vi "log.vi"(9 "响应":string, 11 "发送":string) -> ()   [LabVIEW 2015]
panel:
  in  "应用程序输入":refnum<vi>
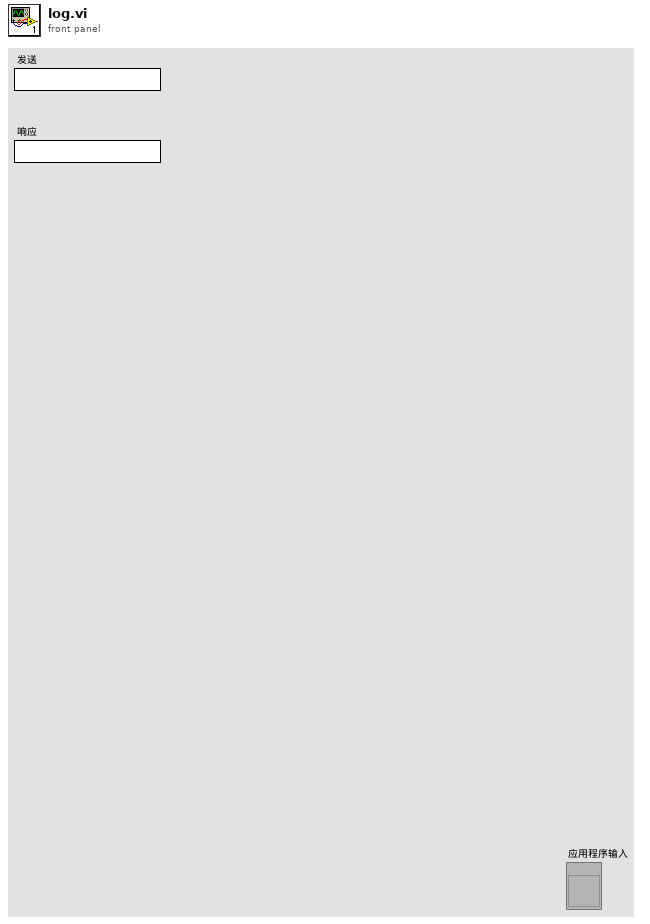
[diagram p1: front panel]
types:
  T1 = enum16{"open", "replace", "create", "open or create", "replace or create", "replace or create with confirmation"}
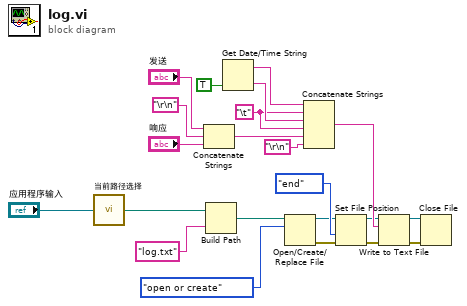
[diagram p0: block diagram]
diagram:
  w9 = "\t"
  n1 = call "当前路径选择.vi"("本应用程序"="应用程序输入") -> ("当前路径"=w3:path)
  n2 = Concatenate Strings("发送", "\r\n", "响应") -> (w5:string)
  n3 = Build Path(base path=w3, name or relative path="log.txt" ("名称或相对路径")) -> (appended path=w1:path)
  n4 = Get Date/Time String(want seconds? (F)=TRUE ("需要秒？(F)")) -> (date string=w11:string, time string=w10:string)  [unwired: 2 in]
  n5 = Open/Create/Replace File(file path (use dialog)=w1, operation (0:open)=T1."open or create" ("操作(0:open)")) -> (refnum out=w16:refnum<file>, error out=w17:errorcluster)  [unwired: 4 in, 1 out]
  n6 = Concatenate Strings(w11, w9, w10, w9, w5, "\r\n") -> (w22:string)
  n7 = Set File Position(refnum=w16, from (0:start)=enum16{"start", "end", "current"}."end" ("自（0:起始）"), error in=w17) -> (refnum out=w18:refnum<file>, error out=w19:errorcluster)  [unwired: 1 in]
  n8 = Write to Text File(file (use dialog)=w18, text=w22, error in=w19) -> (refnum out=w15:refnum<file>, error out=w14:errorcluster)  [unwired: 1 in, 1 out]
  n9 = Close File(refnum=w15, error in=w14) -> ()  [unwired: 2 out]
